vi "2-4-1 LabVIEW WebSocket TX.vi"() -> ()   [LabVIEW 2020]
uses:
  <vilib>/addons/WebSockets-API-master/WebSockets/WebSocket Client/WebSocket Client.lvclass
  C:/Program Files (x86)/National Instruments/LabVIEW 2020/vi.lib/addons/WebSockets-API-master/WebSockets/WebSocket/WebSocket.lvclass
  <vilib>/addons/WebSockets-API-master/WebSockets/WebSocket/WebSocket.lvclass
panel:
  in  "Stop":bool
  out "connection error?":bool
  in  "sensor_data":T1={"temperature"=82.3, "pressure"=1.103, "motor_on"=FALSE, "status"="RUNNING", "timestamp"="2026-07-26 14:32:05"}
  out "connect?":bool
  in  "WebSockets URL":string="ws://echo.websocket.org"
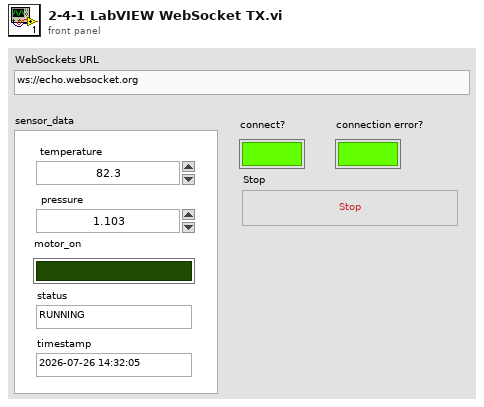
[diagram p1: front panel]
types:
  T1 = cluster{"temperature":dbl, "pressure":dbl, "motor_on":bool, "status":string, "timestamp":string}
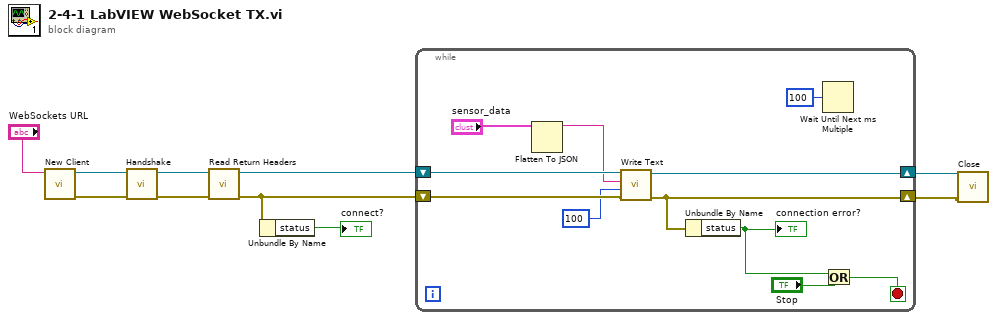
[diagram p0: block diagram]
diagram:
  n1 = call <vilib>:"New Client.vi"("WebSocket URL"="WebSockets URL") -> ("error out"=w10:errorcluster, "WebSocket Client out"=w8:refnum<class "WebSocket Client.lvclass">)  [unwired: 9 in]
  n2 = call-dynamic "Handshake.vi"("error in (no error)"=w10, "WebSocket Client in"=w8) -> ("error out"=w7:errorcluster, "WebSocket Client out"=w6:refnum<class "WebSocket Client.lvclass">)  [unwired: 8 in]
  n3 = call <vilib>:"Read Return Headers.vi"("error in (no error)"=w7, "WebSocket in"=w6) -> ("error out"=w4:errorcluster, "WebSocket out"=w5:refnum<class "WebSocket Client.lvclass">)  [unwired: 7 in, 1 out]
  n4 = Unbundle By Name(w4) -> ("status"=→"connect?":bool)
  n5 = while {
    shift-right: [w18] -> w2
    shift-left: w5 -> [w20]
    shift-right: [w17] -> w1
    shift-left: w4 -> [w19]
    stop <- w14 stop-if-true
    n6 = Flatten To JSON(anything="sensor_data") -> (JSON string=w13:string)  [unwired: 2 in, 1 out]
    n7 = call-dynamic "Write Text.vi"("error in (no error)"=w19, "timeout ms (5000)"=100, "String Data"=w13, "WebSocket in"=w20) -> ("error out"=w17:errorcluster, "WebSocket out"=w18:refnum<class "WebSocket Client.lvclass">)  [unwired: 6 in]
    n8 = Unbundle By Name(w17) -> ("status"=w16:bool)
    "connection error?" <- w16
    n9 = Wait Until Next ms Multiple(millisecond multiple=u32 100) -> ()  [unwired: 1 out]
    n10 = Or(x=w16, y="Stop") -> (x .or. y?=w14:bool)
  }
  n11 = call-dynamic "Close.vi"("error in (no error)"=w1, "WebSocket in"=w2) -> ()  [unwired: 9 in, 1 out]
